vi "Initialize.vi"(8 "error in (no error)":errorcluster caption="错误输入（无错误）", 10 "Status":string, 11 "User Interface 输入":refnum<class "User Interface.lvclass">) -> (0 "error out":errorcluster caption="错误输出", 3 "User Interface 输出":refnum<class "User Interface.lvclass">)   [LabVIEW 2018, in "MainInterface.lvlib" / "User Interface.lvclass"]
uses:
  User Interface.lvclass
  Module Information.ctl
  User Interface.lvclass/User Interface.ctl
  ModuleInterface/ModuleInterface.lvlib
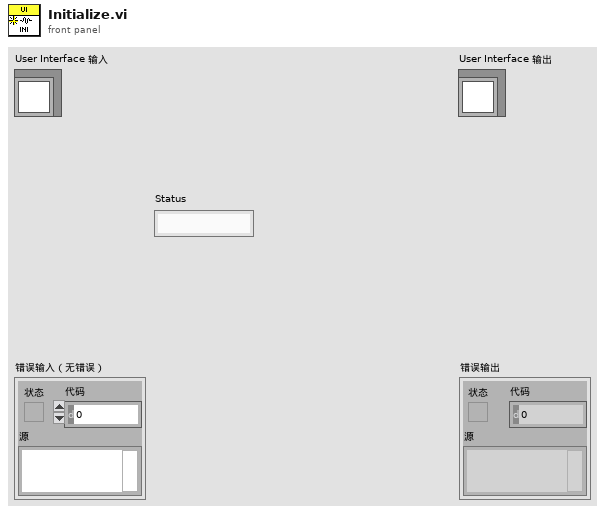
[diagram p1: front panel]
types:
  T1 = typedef "MainInterface.lvlib/User Interface.lvclass/Module Information.ctl" = cluster{"Module ID":i32, "Module Name":string}
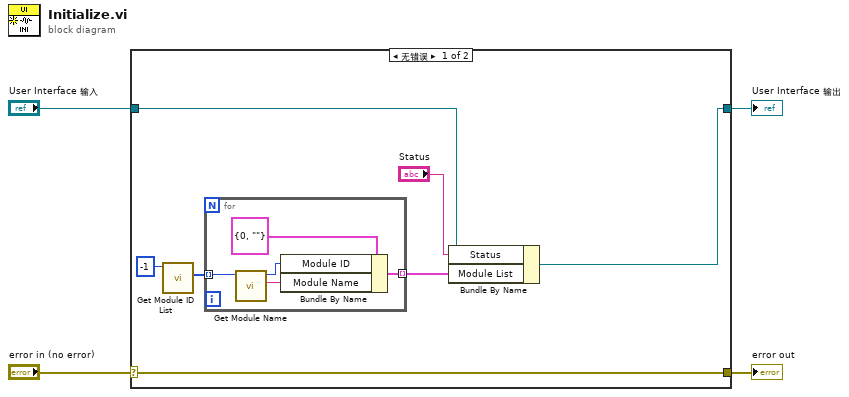
[diagram p0: block diagram]
diagram:
  n1 = case shown="无错误" "error in (no error)" {
    selector: "error in (no error)" -> [w10 w18]
    tunnel: [w10 w18] -> w3
    tunnel: [w6 w17] -> w1
    tunnel: "User Interface 输入" -> [w11 w17]
    frame No Error {
      n2 = call "Get Module ID List.vi"("Module ID"=-1) -> ("Module ID List"=w8:i32[])  [unwired: 8 in, 2 out]
      n3 = for {
        tunnel: w8 -> [w15] mode=indexing
        tunnel: [w12] -> w7 mode=indexing
        n4 = call "Get Module Name.vi"("Module ID"=w15) -> ("Module Name"=w13:string, "Module ID"=w14:i32)  [unwired: 7 in, 2 out]
        n5 = Bundle By Name(cluster=T1 {"Module ID"=0, "Module Name"=""} ("Module Info"), "Module ID"=w14, "Module Name"=w13) -> (w12:T1)
      }
      n6 = Bundle By Name(cluster=w11, "Status"="Status", "Module List"=w7) -> (w6:refnum<class "User Interface.lvclass">)
    }
    frame Error {
    }
  }
  "error out" <- w3
  "User Interface 输出" <- w1
